vi "PalmSense Save Config File.vi"() -> (0 "error out":errorcluster)   [LabVIEW 2020]
uses:
  support/PCT FGV CMD.ctl
  <vilib>/Utility/config.llb/Write Key (Double).vi
  <vilib>/Utility/config.llb/NI_LVConfig.lvlib
  <vilib>/Utility/config.llb/Write Key (String).vi
  <vilib>/regexp/Match Regular Expression.xnode
  <vilib>/Utility/config.llb/Write Key (Path).vi
  <vilib>/Utility/config.llb/Write Key (Boolean).vi
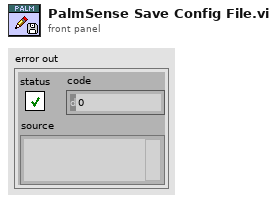
[diagram p1: front panel]
types:
  T1 = typedef "PCT FGV CMD.ctl" = enum16{"INIT", "GET", "SET"}
  T2 = typedef "NI_LVConfig.lvlib/Config Data RefNum.ctl" = refnum<k1>
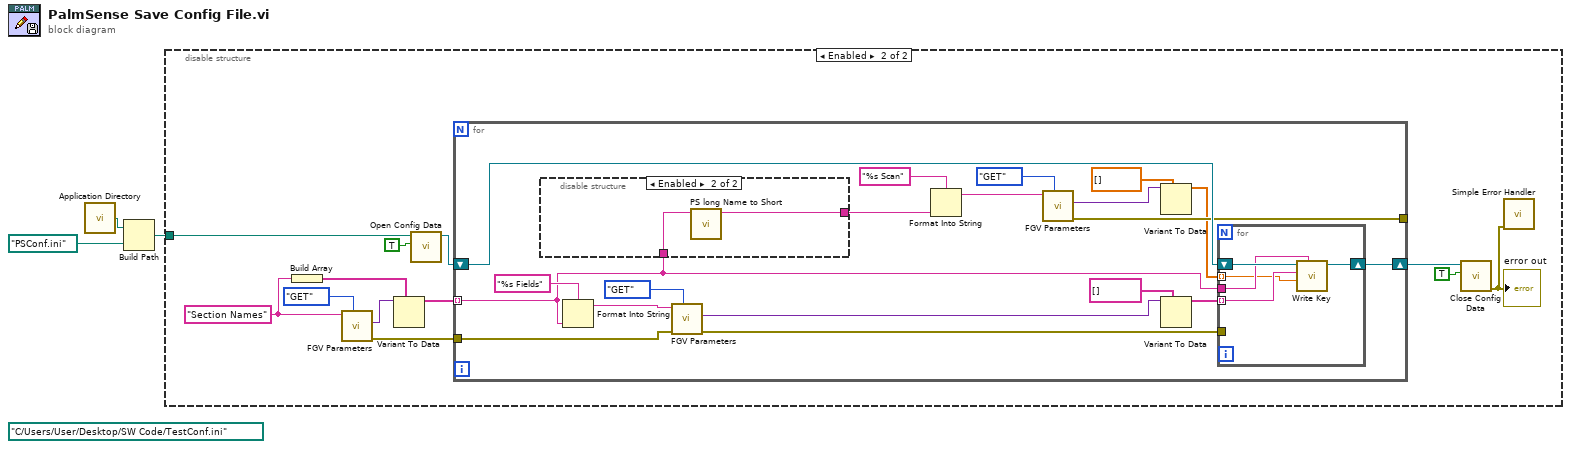
[diagram p0: block diagram]
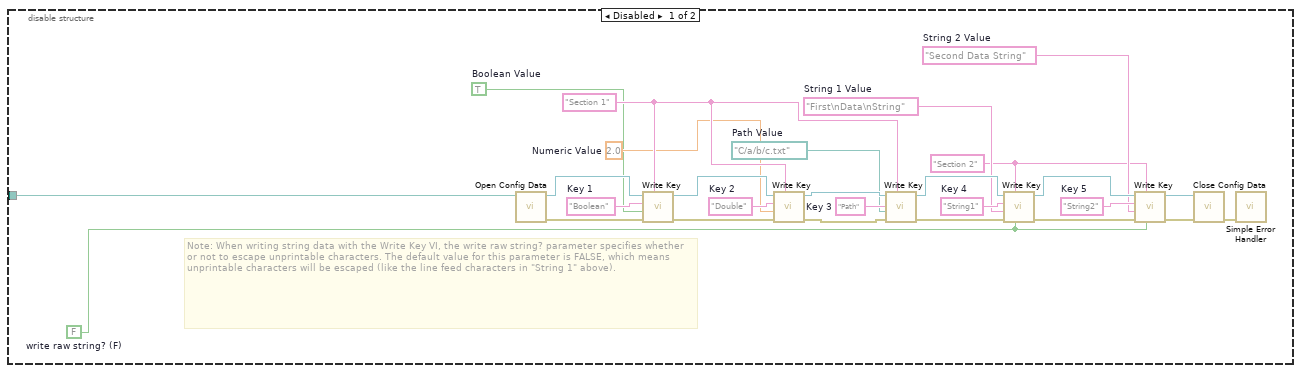
[diagram p2: hidden frame]
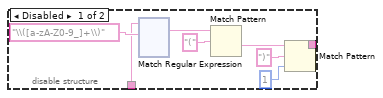
[diagram p3: hidden frame]
diagram:
  (unwired) path "C:/Users/User/Desktop/SW Code/TestConf.ini" ("configuration file path")
  n1 = call <vilib>:"Application Directory.vi"() -> ("Application Directory"=w3:path)
  n2 = Build Path(base path=w3, name or relative path=path "PSConf.ini" ("configuration file path")) -> (appended path=w1:path)
  n3 = disable-structure shown="Enabled" {
    disable-tunnel: w1 -> [w4 w39]
    frame Disabled {
      w12 = "Second Data String"  # String 2 Value
      w13 = "First\nData\nString"  # String 1 Value
      w8 = path "C:/a/b/c.txt"  # Path Value
      w7 = 2.0  # Numeric Value
      w6 = TRUE  # Boolean Value
      w5 = FALSE  # write raw string? (F)
      w14 = "String2"  # Key 5
      w15 = "String1"  # Key 4
      w16 = "Path"  # Key 3
      w17 = "Double"  # Key 2
      w18 = "Boolean"  # Key 1
      w9 = "Section 2"
      w10 = "Section 1"
      # "Note: When writing string data with the Write Key VI, the write raw string? parameter specifies whether or not to escape unprintable characters. The default value for this parameter is FALSE, which means unprintable characters will be escaped (like the line feed characters in \"String 1\" above)."
      n4 = call <vilib>:"Open Config Data.vi"("configuration file path"=w4) -> ("error out"=w24:errorcluster, "refnum"=w30:T2)  [unwired: 2 in, 7 out]
      n5 = call-poly <vilib>:"Write Key.vi"("section"=w10, "error in (no error)"=w24, "value"=w6, "key"=w18, "refnum"=w30) -> ("error out"=w23:errorcluster, "refnum out"=w29:T2)  [unwired: 5 out]
      n6 = call-poly <vilib>:"Write Key.vi"("section"=w10, "error in (no error)"=w23, "value"=w7, "key"=w17, "refnum"=w29) -> ("error out"=w22:errorcluster, "refnum out"=w28:T2)  [unwired: 3 in, 2 out]
      n7 = call-poly <vilib>:"Write Key.vi"("section"=w10, "error in (no error)"=w22, "value"=w8, "key"=w16, "refnum"=w28) -> ("error out"=w21:errorcluster, "refnum out"=w27:T2)  [unwired: 5 out]
      n8 = call-poly <vilib>:"Write Key.vi"("write raw string? (F)"=w5, "section"=w9, "error in (no error)"=w21, "value"=w13, "key"=w15, "refnum"=w27) -> ("error out"=w20:errorcluster, "refnum out"=w26:T2)  [unwired: 4 out]
      n9 = call-poly <vilib>:"Write Key.vi"("write raw string? (F)"=w5, "section"=w9, "error in (no error)"=w20, "value"=w12, "key"=w14, "refnum"=w26) -> ("error out"=w19:errorcluster, "refnum out"=w25:T2)  [unwired: 4 out]
      n10 = call <vilib>:"Close Config Data.vi"("error in (no error)"=w19, "refnum"=w25) -> ("error out"=w11:errorcluster)  [unwired: 1 in, 8 out]
      n11 = call <vilib>:"Simple Error Handler.vi"("error in (no error)"=w11) -> ()  [unwired: 1 in, 8 out]
    }
    frame Enabled {
      w34 = "Section Names"
      n12 = Build Array(w34) -> (w33:string[])
      n13 = call "FGV Parameters.vi"("CMD"=PCT_FGV_CMD."GET", "Key"=w34) -> ("error out"=w35:errorcluster, "output"=w32:variant)  [unwired: 7 in, 1 out]
      n14 = Variant To Data(type=w33, Variant=w32) -> (data=w31:string[])  [unwired: 1 in, 1 out]
      n15 = call <vilib>:"Open Config Data.vi"("create file if necessary (T)"=TRUE ("create file if necessary? (T)"), "configuration file path"=w39) -> ("refnum"=w38:T2)  [unwired: 7 in, 2 out]
      n16 = for {
        tunnel: w31 -> [w53] mode=indexing
        shift-right: [w60] -> w37
        shift-left: w38 -> [w61]
        tunnel: w35 -> [w58]
        tunnel: [w49] -> _
        n17 = disable-structure shown="Enabled" {
          disable-tunnel: w53 -> [w63 w185]
          disable-tunnel: [w62 w184] -> w52
          frame Disabled {
            n18 = xnode "Match Regular Expression"("input string"=w63, "regular expression"="\\([a-zA-Z0-9_]+\\)") -> ("whole match"=w66:string)  [unwired: 4 in, 4 out]
            n19 = Match Pattern(string=w66, regular expression="(") -> (after substring=w64:string)  [unwired: 1 in, 3 out]
            n20 = Match Pattern(string=w64, regular expression=")", offset (0)=1) -> (before substring=w62:string)  [unwired: 3 out]
          }
          frame Enabled {
            n21 = call "PS long Name to Short.vi"("String"=w185) -> ("whole match"=w184:string)  [unwired: 10 in]
          }
        }
        n22 = Format Into String(format string="%s Fields", w53) -> (resulting string=w56:string)  [unwired: 2 in, 1 out]
        n23 = call "FGV Parameters.vi"("CMD"=PCT_FGV_CMD."GET", "error in (no error)"=w58, "Key"=w56) -> ("error out"=w55:errorcluster, "output"=w45:variant)  [unwired: 6 in, 1 out]
        n24 = Format Into String(format string="%s Scan" ("Key"), w52) -> (resulting string=w50:string)  [unwired: 2 in, 1 out]
        n25 = call "FGV Parameters.vi"("CMD"=PCT_FGV_CMD."GET", "Key"=w50) -> ("error out"=w49:errorcluster, "output"=w47:variant)  [unwired: 7 in, 1 out]
        n26 = Variant To Data(type=dbl[] [] ("number"), Variant=w47) -> (data=w46:dbl[])  [unwired: 1 in, 1 out]
        n27 = Variant To Data(type=string[] [], Variant=w45) -> (data=w43:string[])  [unwired: 1 in, 1 out]
        n28 = for {
          tunnel: w53 -> [w188]
          tunnel: w43 -> [w187] mode=indexing
          shift-right: [w189] -> w60
          shift-left: w61 -> [w190]
          tunnel: w55 -> [_]
          tunnel: w46 -> [w186] mode=indexing
          n29 = call-poly <vilib>:"Write Key.vi"("section"=w188, "value"=w186, "key"=w187, "refnum"=w190) -> ("refnum out"=w189:T2)  [unwired: 5 in, 2 out]
        }
      }
      n30 = call <vilib>:"Close Config Data.vi"("write file if changed (T)"=TRUE ("write configuration file? (T)"), "refnum"=w37) -> ("error out"=w40:errorcluster)  [unwired: 1 in, 8 out]
      "error out" <- w40
      n31 = call <vilib>:"Simple Error Handler.vi"("error in (no error)"=w40) -> ()  [unwired: 1 in, 8 out]
    }
  }
